vi "DMR_GetImageRequestBufferData.vi"(1 "driver handle IN":i32, 4 "request number IN":i32) -> (10 "pData OUT":i32, 11 "width OUT":i32, 12 "pixel format OUT":T1(ring), 13 "height OUT":i32, 14 "driver handle OUT":i32, 15 "request number OUT":i32, 16 "bytes per pixel OUT":i32, 17 "channel count OUT":i32, 18 "size OUT":i32, 19 "error code OUT":i32)   [LabVIEW 2016]
doc: "Returns information about the image associated with the desired request.\n\nAlways call this function to receive the up to date data for the current request and do NOT use this data for any other request!\n\nThe 'request number IN' parameter can be obtained from the DMR_ImageRequestWaitFor VI.\n\nSee also:\nDMR_GetImageRequestBufferChannelData\n\nThe 'error code OUT' terminal will deliver 0 if successful or a negative error code otherwise. A list of valid error codes and their meaning can be found in the manual about this interface."
uses:
  mvDeviceManager.dll
panel:
  # "OUTPUT"
  # "INPUT"
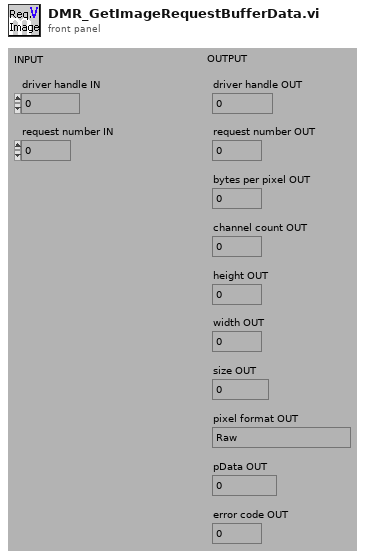
[diagram p1: front panel]
types:
  T1 = enum16{"Raw", "Mono8", "Mono16", "RGBx888Packed", "YUV422Packed", "RGBx888Planar", "Mono10", "Mono12", "Mono14", "RGB888Packed", "YUV444Planar", "Mono32", "YUV422Planar", "RGB101010Packed", "RGB121212Packed", "RGB141414Packed", "RGB161616Packed", "YUV422_UYVYPacked", "Mono12Packed_V2", "Reserved1", "YUV422_10Packed", "YUV422_UYVY_10Packed", "BGR888Packed", "BGR101010Packed_V2", "YUV444_UYVPacked", "YUV444_UYV_10Packed", "YUV444Packed", "YUV444_10Packed"}
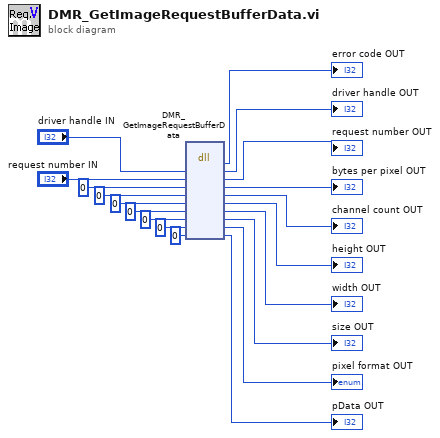
[diagram p0: block diagram]
diagram:
  n1 = dll-call lib="mvDeviceManager.dll" fn="DMR_GetImageRequestBufferData"("hDrv"="driver handle IN", "requestNr"="request number IN", "pBytesPerPixel"=0, "pChannelCount"=0, "pHeight"=0, "pWidth"=0, "pSize"=0, "pPixelFormat"=0, "pData"=0) -> (→"error code OUT":i32, "hDrv"=→"driver handle OUT":i32, "requestNr"=→"request number OUT":i32, "pBytesPerPixel"=→"bytes per pixel OUT":i32, "pChannelCount"=→"channel count OUT":i32, "pHeight"=→"height OUT":i32, "pWidth"=→"width OUT":i32, "pSize"=→"size OUT":i32, "pPixelFormat"=→"pixel format OUT":i32, "pData"=→"pData OUT":i32)  [unwired: 3 in, 2 out]
